vi "Calculate Distance.vi"(6 "Robot Calibration Cluster":T1={"Camera Height on robot (in)"=34.5, "Camera Angle on the robot (deg)"=28.3, "Slope"=0.946, "Offset"=10.775} {"Offset" format="%#_13g"; "Slope" format="%#_13g"; "Camera Angle on the robot (deg)" format="%#_13g"; "Camera Height on robot (in)" format="%#_13g"}, 8 "Height to center of target from floor (hp (in))":dbl=98.25 format="%#_13g", 9 "Screen resolution pixels Height (Ry)":dbl=360.0 format="%#_13g", 11 "Middle of target from 0,0 (pixels)":dbl=178.5 format="%#_13g") -> (3 "Distance from target (in)":dbl=116.40675998176638 format="%.2f")   [LabVIEW 2023]
panel:
  in  "Camera FOV Top to BottomView Angle (deg)":dbl=49.0 format="%#_13g"
  # "These Items are inputs"
  # "These items should only have to be figured out one time each season unless the camera mounting changes"
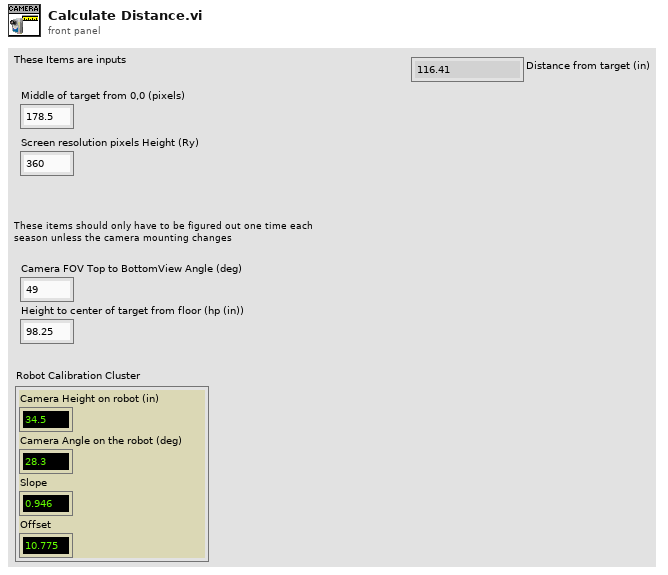
[diagram p1: front panel]
types:
  T1 = cluster{"Camera Height on robot (in)":dbl, "Camera Angle on the robot (deg)":dbl, "Slope":dbl, "Offset":dbl}
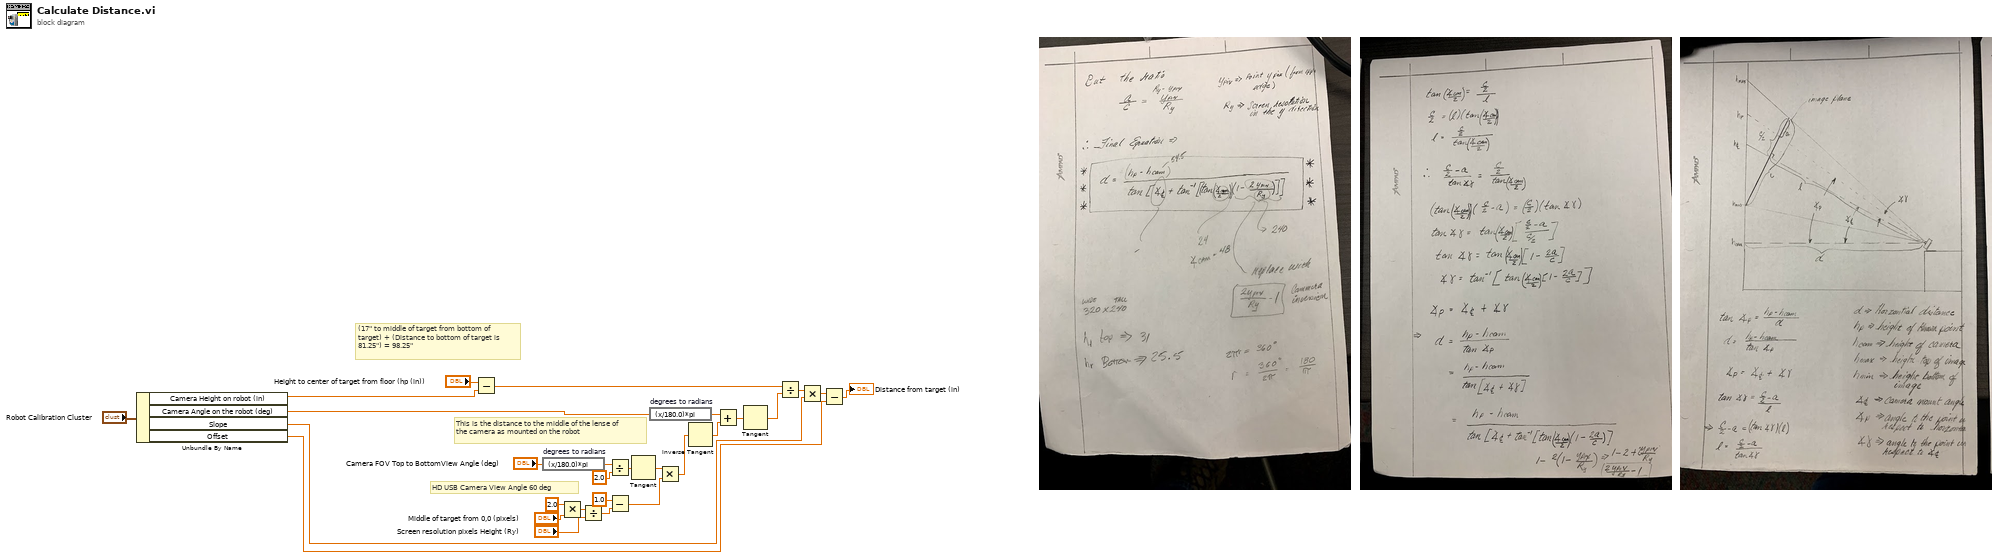
[diagram p0: block diagram]
diagram:
  # "HD USB Camera View Angle 60 deg"
  # "(17\" to middle of target from bottom of target) + (Distance to bottom of target is 81.25\") = 98.25\""
  # "This is the distance to the middle of the lense of the camera as mounted on the robot"
  n1 = Unbundle By Name("Robot Calibration Cluster") -> ("Camera Height on robot (in)"=w4:dbl, "Camera Angle on the robot (deg)"=w3:dbl, "Slope"=w2:dbl, "Offset"=w1:dbl)
  n2 = Subtract(x="Height to center of target from floor (hp (in))", y=w4) -> (x-y=w26:dbl)
  n3 = expression code="(x/180.0)*pi" "degrees to radians"("Camera FOV Top to BottomView Angle (deg)") -> (w12:dbl)
  n4 = Multiply(x=2.0, y="Middle of target from 0,0 (pixels)") -> (x*y=w21:dbl)
  n5 = Divide(x=w21, y="Screen resolution pixels Height (Ry)") -> (x/y=w19:dbl)
  n6 = Divide(x=w12, y=2.0) -> (x/y=w17:dbl)
  n7 = Subtract(x=1.0, y=w19) -> (x-y=w15:dbl)
  n8 = Tangent(1:w17) -> (0:w16:dbl)
  n9 = expression code="(x/180.0)*pi" "degrees to radians"(w3) -> (w11:dbl)
  n10 = Multiply(x=w16, y=w15) -> (x*y=w14:dbl)
  n11 = Inverse Tangent(1:w14) -> (0:w25:dbl)
  n12 = Add(x=w11, y=w25) -> (x+y=w10:dbl)
  n13 = Tangent(1:w10) -> (0:w9:dbl)
  n14 = Divide(x=w26, y=w9) -> (x/y=w7:dbl)
  n15 = Multiply(x=w7, y=w2) -> (x*y=w8:dbl)
  n16 = Subtract(x=w8, y=w1) -> (x-y=→"Distance from target (in)":dbl)
